vi "create.orderbook.commands.for.testing.vi"(11 "OrderBook.Commands.in":T1[](array[typedef])=[{"OrderBook Command.Type"=enum."AddOrder", "Side (U8)"=66, "Order Id (U64)"=48, "Quantity (U32)"=20000, "Symbol (U64)"=4702127773838221344, "Price (U64)"=9050, "Executed Quantity (U32)"=0, "Canceled Quantity (U32)"=0, "Remaining Quantity (U32)"=0, "Seconds (U64)"=0, "Nanoseconds (U64)"=0}] {"Side (U8)" format="%.0x"; "Order Id (U64)" format="%.0x"; "Symbol (U64)" format="%.0x"}) -> (3 "Words.Out":u64[](array[numeric])=[1, 66, 48, 20000, 4702127773838221344, 9050, 0, 0, 0, 0, 0, 0, 0, 0, 0, 0, 2, 66, 48, 0, 0, 9050, 200, 0, 0, 0, 0, 0, 0, 0, 0, 0, 5, 66, 48, 1400, 6076284164848492576, 9050, 0, 0, 0, 0, 0, 0, 0, 0, 0, 0] format="%.0x")   [LabVIEW 2022 SP3]
uses:
  fpga/common/orderbook.command.ctl
  fpga/common/orderbook.command.type.ctl
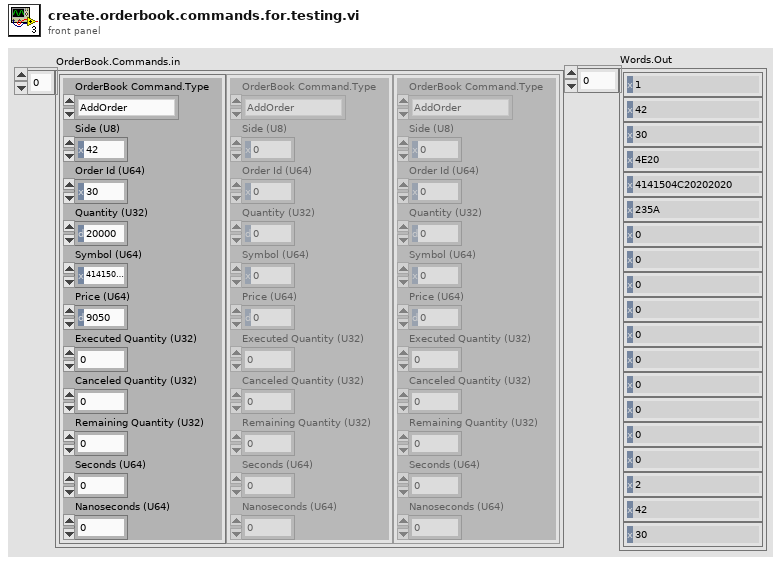
[diagram p1: front panel]
types:
  T1 = typedef "orderbook.command.ctl" = cluster{"OrderBook Command.Type":T2, "Side (U8)":u8, "Order Id (U64)":u64, "Quantity (U32)":u32, "Symbol (U64)":u64, "Price (U64)":u64, "Executed Quantity (U32)":u32, "Canceled Quantity (U32)":u32, "Remaining Quantity (U32)":u32, "Seconds (U64)":u64, "Nanoseconds (U64)":u64}
  T2 = typedef "orderbook.command.type.ctl" = enum16{"Time", "AddOrder", "OrderExecuted", "OrderExecutedAtPrice", "ReduceSize", "ModifyOrder", "DeleteOrder", "Get.State", "Get.All.Orders", "Get.Top"}
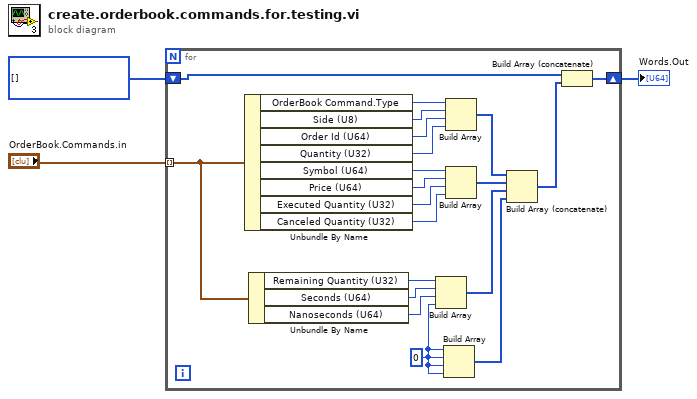
[diagram p0: block diagram]
diagram:
  n1 = for {
    tunnel: "OrderBook.Commands.in" -> [w23] mode=indexing
    shift-right: [w5] -> w1
    shift-left: u64[] [] -> [w7]
    w12 = u64 0 ("element")
    n2 = Unbundle By Name(w23) -> ("OrderBook Command.Type"=w22:T2, "Side (U8)"=w21:u8, "Order Id (U64)"=w20:u64, "Quantity (U32)"=w19:u32, "Symbol (U64)"=w18:u64, "Price (U64)"=w17:u64, "Executed Quantity (U32)"=w16:u32, "Canceled Quantity (U32)"=w15:u32)
    n3 = Unbundle By Name(w23) -> ("Remaining Quantity (U32)"=w14:u32, "Seconds (U64)"=w13:u64, "Nanoseconds (U64)"=w4:u64)
    n4 = Build Array(w14, w13, w4, w12) -> (w9:u64[])
    n5 = Build Array(w12, w12, w12, w12) -> (w8:u64[])
    n6 = Build Array(w22, w21, w20, w19) -> (w11:u64[])
    n7 = Build Array(w18, w17, w16, w15) -> (w10:u64[])
    n8 = Build Array (concatenate)(w11, w10, w9, w8) -> (w6:u64[])
    n9 = Build Array (concatenate)(w7, w6) -> (w5:u64[])
  }
  "Words.Out" <- w1
